vi "Multiple Relay set.vi"() -> (2 "Command":string)   [LabVIEW 2025]
panel:
  in  "Array":T1(array[ring])
  in  "x":dbl format="%#_13g"
  out "Array 2":string[][](array[string])
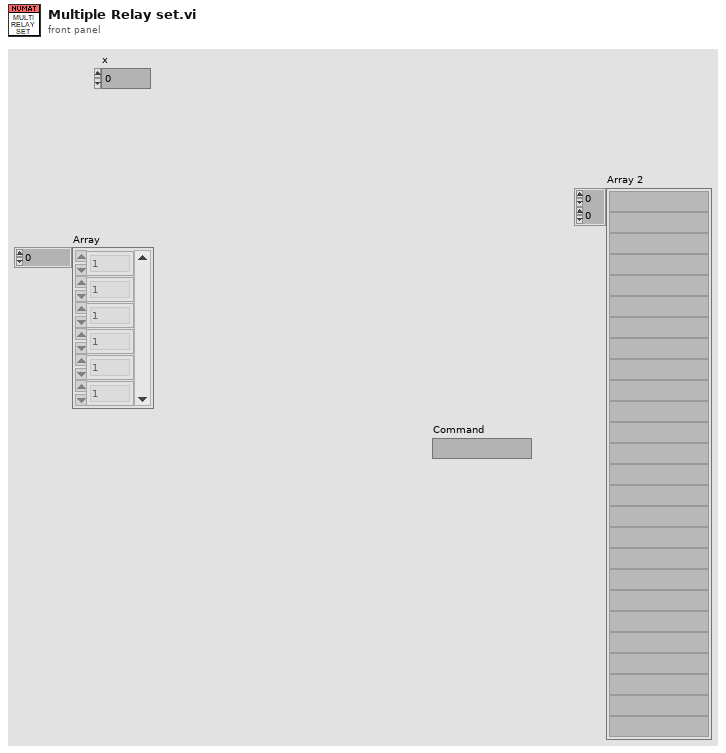
[diagram p1: front panel]
types:
  T1 = enum16{"1", "2", "3", "4", "5", "6", "7", "8", "9", "10", "11", "12", "13", "14", "15", "16", "17", "18", "19", "20", "21", "22", "23", "24", "25", "26", "27", "28", "29", "30", "31", "32"}[]
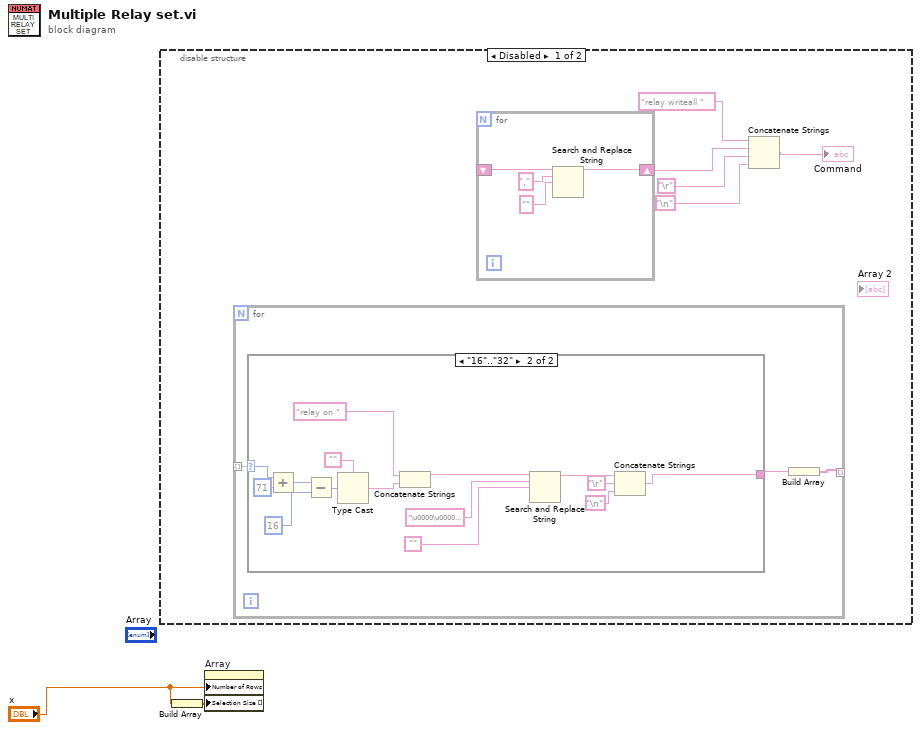
[diagram p0: block diagram]
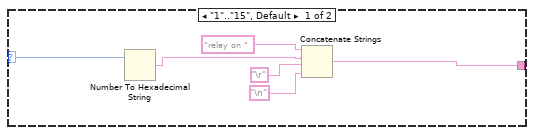
[diagram p2: hidden frame]
diagram:
  n1 = disable-structure shown="Disabled" {
    frame Disabled {
      n2 = for {
        tunnel: _ -> [w11] mode=indexing
        tunnel: [w10] -> w3 mode=indexing
        n3 = case shown="\"16\"..\"32\"" w11 {
          selector: w11 -> [w17 w18]
          tunnel: [w12 w19] -> w9
          frame "1".."15", Default {
            n4 = Number To Hexadecimal String(2:w17) -> (0:w13:string)  [unwired: 1 in]
            n5 = Concatenate Strings("relay on " ("initial string"), w13, "\r", "\n") -> (w12:string)
          }
          frame "16".."32" {
            n6 = Add(x=w18, y=71) -> (x+y=w31:i32)
            n7 = Subtract(x=w31, y=16) -> (x-y=w29:i32)
            n8 = Type Cast(type="", x=w29) -> (*(type *) &x=w27:string)
            n9 = Concatenate Strings("relay on " ("initial string"), w27) -> (w23:string)
            n10 = Search and Replace String(input string=w23, search string="\u0000\u0000\u0000" ("Command"), replace string="") -> (result string=w22:string)  [unwired: 5 in, 3 out]
            n11 = Concatenate Strings(w22, "\r", "\n" ("string")) -> (w19:string)
          }
        }
        n12 = Build Array(w9) -> (w10:string[])
      }
      n13 = for {
        shift-right: [w35] -> w5
        shift-left: _ -> [w36]
        n14 = Search and Replace String(input string=w36, search string=",", replace string="" ("replace string (\"\")")) -> (result string=w35:string)  [unwired: 5 in, 3 out]
      }
      n15 = Concatenate Strings("relay writeall " ("Command"), w5, "\r", "\n") -> (→"Command":string)
    }
    frame Enabled {
    }
  }
  n16 = Build Array("x") -> (w1:dbl[])
  n17 = property on="Array" class="Arr (strict)"("Number of Rows"="x", "Selection Size []"=w1) -> ()  [unwired: 2 in, 2 out]
